vi "connection test.vi"() -> ()   [LabVIEW 2015]
uses:
  <vilib>/Instr/_visa.llb/VISA Configure Serial Port (Instr).vi
panel:
  in  "Query?":bool
  in  "VISA resource name":refnum<visa-resource-name>="COM11"
  out "Config error":errorcluster
  out "writting count":u32
  out "reading count":u32
  out "reading error":errorcluster
  out "read buffer":string
  in  "write buffer":string
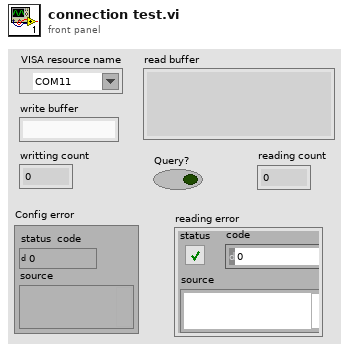
[diagram p1: front panel]
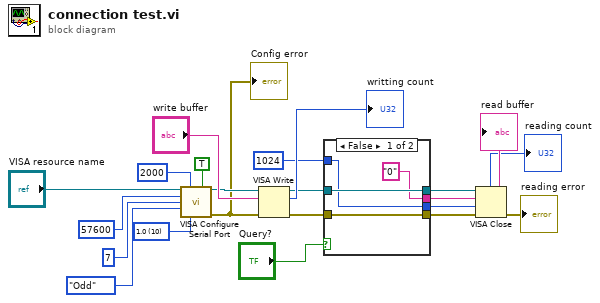
[diagram p0: block diagram]
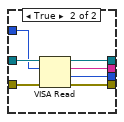
[diagram p2: hidden frame]
diagram:
  w9 = u16 10 items=["1.0"=10, "1.5"=15, "2.0"=20] ("stop bits (10: 1 bit)")
  n1 = call-poly "VISA Configure Serial Port"("VISA resource name"="VISA resource name", "timeout (10sec)"=u32 2000, "Enable Termination\nChar (T)"=TRUE ("Enable Termination\nChar (T)"), "baud rate (9600)"=u32 57600, "data bits (8)"=u16 7, "parity (0:none)"=enum16{"None", "Odd", "Even", "Mark", "Space"}."Odd", "stop bits (10: 1 bit)"=w9) -> ("VISA resource name out"=w13:refnum<visa-resource-name>, "error out"=w12:errorcluster)  [unwired: 7 in]
  "Config error" <- w12
  n2 = VISA Write(VISA resource name=w13, write buffer="write buffer", error in (no error)=w12) -> (VISA resource name out=w5:refnum<visa-resource-name>, return count=→"writting count":u32, error out=w6:errorcluster)
  n3 = case shown="False" "Query?" {
    tunnel: [w24 w31] -> w20
    tunnel: ["0" ("read buffer") w30] -> w19
    tunnel: [w23 w29] -> w18
    tunnel: [w22 w28] -> w16
    tunnel: w6 -> [w23 w27]
    tunnel: w5 -> [w24 w26]
    tunnel: u32 1024 ("byte count") -> [w22 w25]
    frame False {
    }
    frame True {
      n4 = VISA Read(VISA resource name=w26, byte count=w25, error in (no error)=w27) -> (VISA resource name out=w31:refnum<visa-resource-name>, read buffer=w30:string, return count=w28:u32, error out=w29:errorcluster)
    }
  }
  "read buffer" <- w19
  "reading count" <- w16
  n5 = VISA Close(VISA resource name=w20, error in (no error)=w18) -> (error out=→"reading error":errorcluster)
